vi "Set Node Dependency.vi"(8 "error in (no error)":errorcluster, 9 "NodeName":string, 10 "Data":variant, 11 "Item Ref in":T1 format="%.0x") -> (0 "error out":errorcluster, 3 "Item Ref out":T1 format="%.0x")   [LabVIEW 2023, in "J1939 Addon System Explorer.lvlib"]
uses:
  J1939 Addon System Explorer.lvlib
  <vilib>/NI VeriStand/Custom Device API/Custom Device Item Ref.ctl
  <vilib>/NI VeriStand/Custom Device API/Set Item Property (Dependent Node Pointer).vi
  <vilib>/NI VeriStand/UI Controls/Single Node Browser/NI_VS UI Single Node Browser.lvlib
  <vilib>/NI VeriStand/Custom Device API/Custom Device API.lvlib
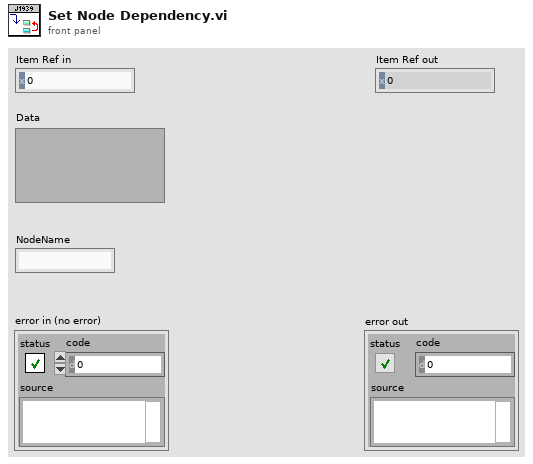
[diagram p1: front panel]
types:
  T1 = typedef "Custom Device API.lvlib/Custom Device Item Ref.ctl" = u64
  T2 = typedef "NI_VS UI Single Node Browser.lvlib/Node Ref.ctl" = refnum<k24>
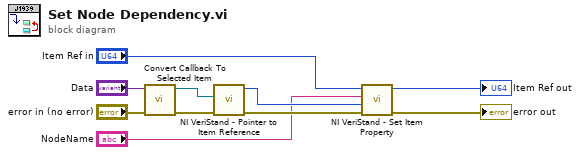
[diagram p0: block diagram]
diagram:
  n1 = call <vilib>:"Convert Callback To Selected Item.vi"("error in"="error in (no error)", "Data"="Data") -> ("error out"=w7:errorcluster, "Selected Item"=w10:T2)  [unwired: 8 in]
  n2 = call <vilib>:"NI VeriStand - Pointer to Item Reference.vi"("error in (no error)"=w7, "Node Pointer"=w10) -> ("error out"=w6:errorcluster, "Item Ref out"=w5:T1)  [unwired: 8 in]
  n3 = call-poly <vilib>:"NI VeriStand - Set Item Property.vi"("error in (no error)"=w6, "Dependent Node Ref"=w5, "Property Name"="NodeName", "Item Ref in"="Item Ref in") -> ("error out"=→"error out":errorcluster, "Item Ref out"=→"Item Ref out":T1)  [unwired: 5 in, 1 out]
